vi "Init Plugins.vi"(8 "error in (no error)":errorcluster, 11 "Execution UI in":refnum<class "Execution UI.lvclass">) -> (0 "error out":errorcluster, 3 "Execution UI out":refnum<class "Execution UI.lvclass">)   [LabVIEW 2020, in "Execution UI.lvclass"]
uses:
  Execution UI.lvclass
  Execution UI.lvclass/Execution UI.ctl
  Framework/Icon Decorator/Icon Decorator.lvclass
  C:/git/astemes-lunit/source/Plugins/Plugin/Plugin.lvclass
  C:/git/astemes-lunit/source/Framework/Result Observer/Result Observer.lvclass
  C:/git/astemes-lunit/source/Framework/Icon Decorator/Icon Decorator.lvclass
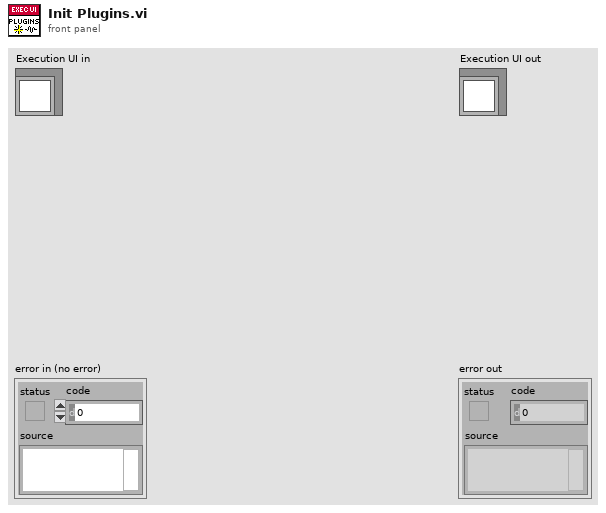
[diagram p1: front panel]
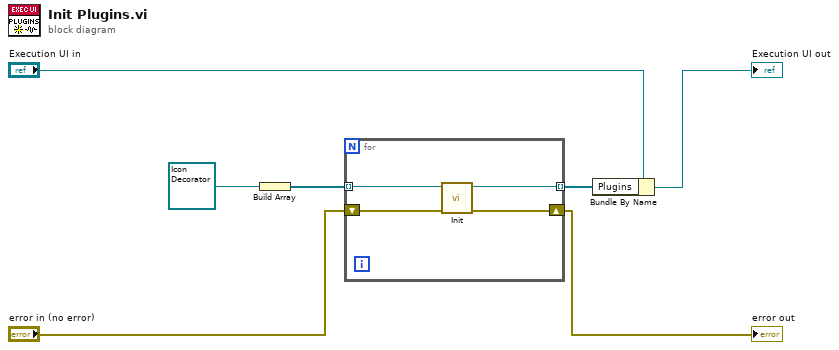
[diagram p0: block diagram]
diagram:
  n1 = Build Array(refnum<class "Icon Decorator.lvclass"> refnum ("Icon Decorator.lvclass")) -> (w5:refnum<class "Icon Decorator.lvclass">[])
  n2 = for {
    tunnel: w5 -> [w11] mode=indexing
    shift-right: [w9] -> w3
    shift-left: "error in (no error)" -> [w10]
    tunnel: [w8] -> w1 mode=indexing
    n3 = call-dynamic "Init.vi"("error in (no error)"=w10, "Icon Decorator In"=w11) -> ("error out"=w9:errorcluster, "Icon Decorator Out"=w8:refnum<class "Icon Decorator.lvclass">)  [unwired: 8 in]
  }
  "error out" <- w3
  n4 = Bundle By Name(cluster="Execution UI in", "Plugins"=w1) -> (→"Execution UI out":refnum<class "Execution UI.lvclass">)
